vi "全局 1.vi"() -> ()   [LabVIEW 2013]
panel:
  in  "波形图 Order":waveform(dbl)(graph)
  in  "边界 Order":dbl[][](array[numeric])
  out "Order 数组":dbl[][](array[numeric])
  out "test passed? 4":bool caption="测试通过？"
  out "Order":cluster{"x0":dbl, "dx":dbl, "Y":dbl[]}[](graph) caption="spectrum"
  out "Waveform":waveform(dbl)
  out "FFT数组":dbl[][](array[numeric])
  out "test passed? 3":bool caption="测试通过？"
  in  "边界 FFT":dbl[][](array[numeric])
  out "FFT":cluster{"x0":dbl, "dx":dbl, "Y":dbl[]}[](graph) caption="spectrum"
  in  "波形图 FFT":waveform(dbl)(graph)
  in  "TCP句柄 2":refnum<k5>
  in  "TCP句柄":refnum<k5>
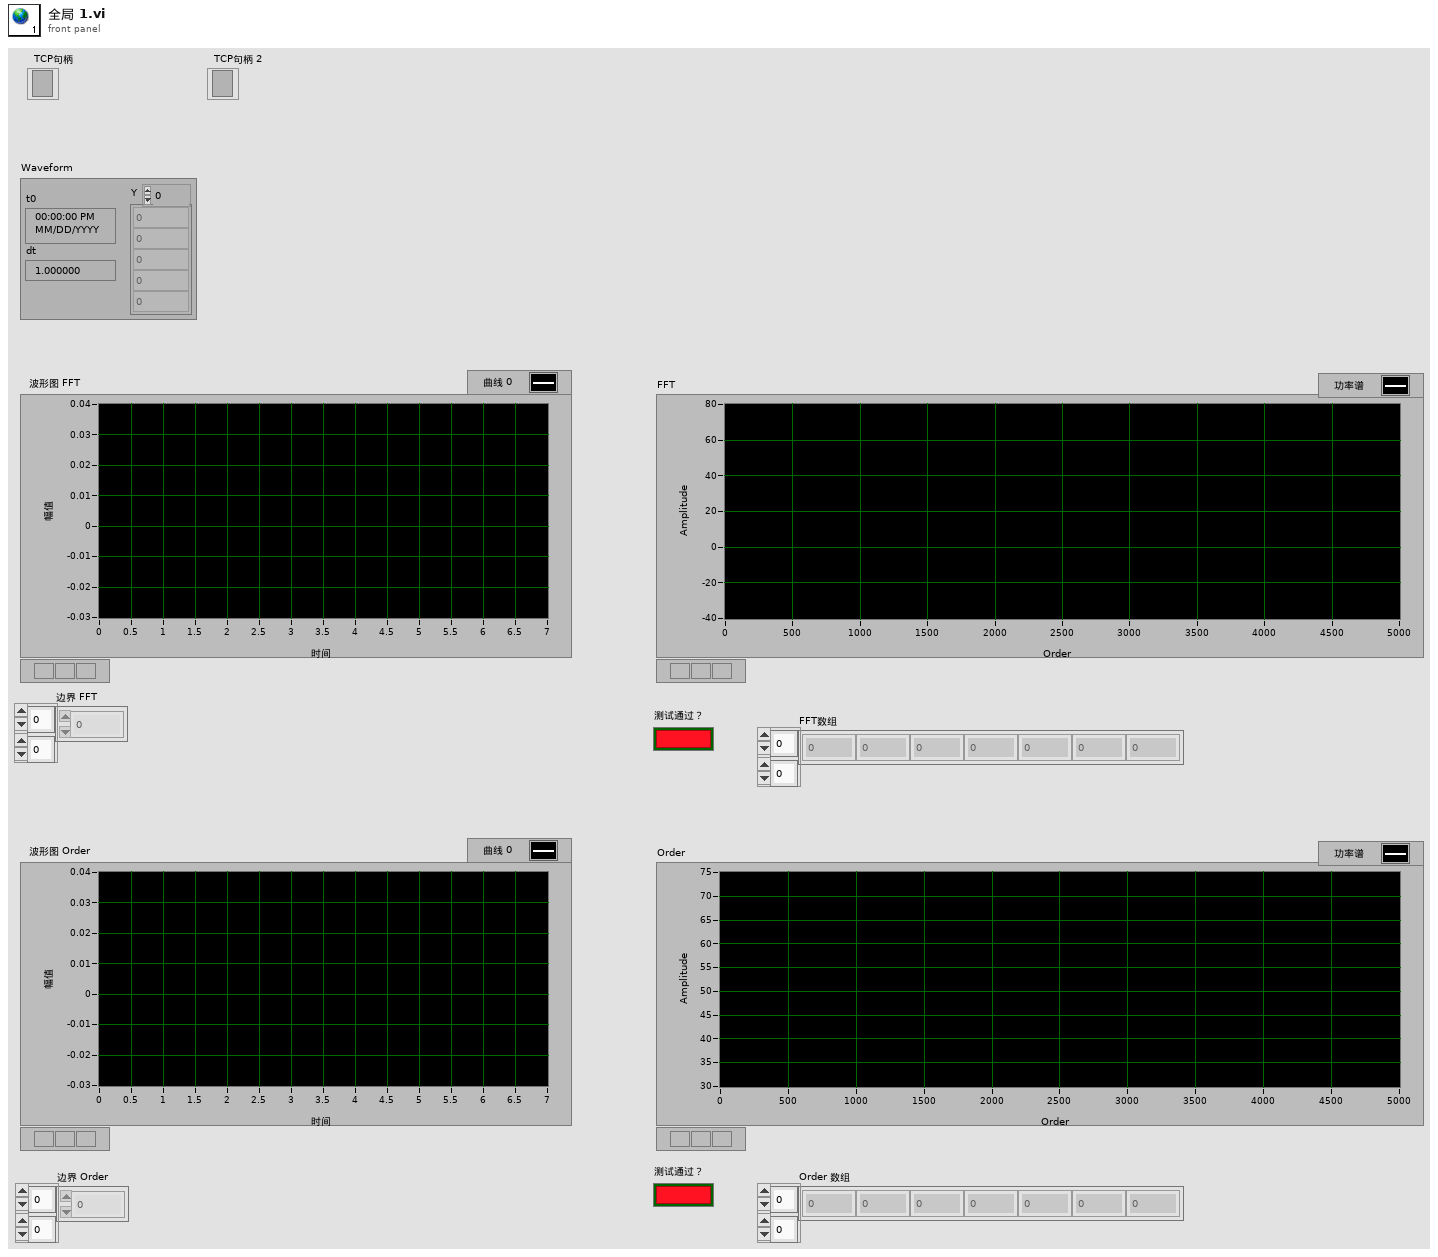
[diagram p1: front panel]
diagram:
